vi "GSI-HVSwitch2.initialize interface.vi"(0 "i ref in":refnum<vi>, 3 "ms timeout (10000)":i32=10000, 5 "error in (no error)":errorcluster) -> (14 "i ref out":refnum<vi>, 17 "timed out":bool, 19 "error out":errorcluster)   [LabVIEW 2014, in "GSI-HVSwitch2.lvlib"]
doc: "Initializes the interface to the instrument. This method must be called prior to communicating with the instrument.\n\nLicense Agreement for this software:\n\nCopyright (C)\nGesellschaft für Schwerionenforschung, GSI\nPlanckstr. 1\n64291 Darmstadt\nGermany\n\nContact: D.Beck@gsi.de \n\nThis program is free software; you can redistribute it and/or modify it under the terms of the GNU General Public License as published by the Free Software Foundation; either version 2 of the license, or (at your option) any later version.\n\nThis program is distributed in the hope that it will be useful, but WITHOUT ANY WARRANTY; without even the implied warranty of MERCHANTABILITY or FITNESS FOR A PARTICULAR PURPOSE. See the GNU General License for more details (http://www.gnu.org).\n\nGesellschaft für Schwerionenforschung, GSI\nPlanckstr. 1, 64291 Darmstadt, Germany\nFor all questions and ideas contact: M.Richter@gsi.de, H.Brand@gsi.de or D.Beck@gsi.de.\nLast update: 17-JUN-2004"
uses:
  GSI-HVSwitch2.lvlib
  CSCore/CSApplicationBaseClasses/PSChannelBase/PSChannelBase.myEventNames.ctl
  CSCore/CSApplicationBaseClasses/PSChannelBase/PSChannelBase.directionType.ctl
  CSCore/CSApplicationBaseClasses/PSChannelBase/PSChannelBase.serviceType.ctl
  CSlibraries/UtilityLib/UtilityLib.valueStatus.ctl
  CSCore/CSApplicationBaseClasses/PSChannelBase/PSChannelBase.lvlib
  CSlibraries/UtilityLib/UtilityLib.lvlib
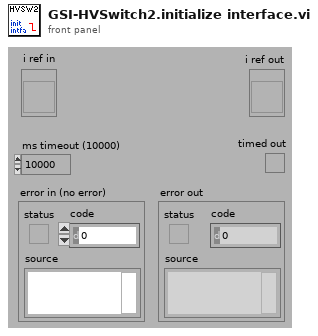
[diagram p1: front panel]
types:
  T1 = typedef "UtilityLib.lvlib/UtilityLib.valueStatus.ctl" = enum16{"no info available", "stand by/off", "on", "warning", "alarm/malfunction", "not implemented", "user action required", "important information", "system default", "control default", "indicator default", "button default"}
  T2 = typedef "PSChannelBase.lvlib/PSChannelBase.serviceType.ctl" = enum16{"onOff", "voltage", "current", "tripCurrent", "rampUpSpeed", "rampDownSpeed", "status"}
  T3 = typedef "PSChannelBase.lvlib/PSChannelBase.directionType.ctl" = enum16{"unknown", "update actual value", "update nominal value", "update both"}
  T4 = typedef "GSI-HVSwitch2.lvlib/GSI-HVSwitch2.i attribute.ctl" = cluster{"SDEX VISA Cluster":T5, "SetVoltage SW0":dbl, "SetVoltage SW1":dbl, "ActTempAmp":dbl, "ActTempPS1":dbl, "ActTempPS2":dbl, "mode":T8, "interfaceInitialized":bool, "serviceIDs":cluster{"nomVoltage0ID":i32, "nomVoltage1ID":i32, "actTempAmpID":i32, "actTempPS1ID":i32, "actTempPS2ID":i32, "modeID":i32}, "usedChannels":i32}
  T5 = typedef "SDEXDriver.lvlib/SDEX.VISA Control.ctl" = cluster{"VISA resource name":refnum<visa-resource-name>, "HEX address":u16, "VISA Timeout Value (1000 ms)":u32, "Lock Timeout (1000 ms)":u32, "semaphore":T6, "Baud rate":u32, "revision":T7, "deviceInfo":string}
  T6 = typedef "Semaphore RefNum" = refnum<k1>
  T7 = typedef "SDEXDriver.lvlib/SDEX.revisionType.ctl" = enum16{"unknown", "hvamp3", "hvswi1", "htrp0", "WDG0"}
  T8 = typedef "GSI-HVSwitch2.lvlib/GSI-HVSwitch2.mode.ctl" = enum16{"unknown", "switch", "stepper"}
  T9 = typedef "PSChannelBase.lvlib/PSChannelBase.myEventNames.ctl" = enum16{"lvmsg://EmergencyOff", "lvmsg://SetOnOff", "lvmsg://GetOnOff", "lvmsg://SetVoltage", "lvmsg://GetVoltage", "lvmsg://SetCurrent", "lvmsg://GetCurrent", "lvmsg://SetTripCurrent", "lvmsg://GetTripCurrent", "lvmsg://SetRampUpSpeed", "lvmsg://GetRampUpSpeed", "lvmsg://SetRampDownSpeed", "lvmsg://GetRampDownSpeed", "lvmsg://SetChannelOnOff", "lvmsg://GetChannelOnOff", "lvmsg://SetChannelVoltage", "lvmsg://GetChannelVoltage", "lvmsg://SetChannelCurrent", "lvmsg://GetChannelCurrent", "lvmsg://SetChannelTripCurrent", "lvmsg://GetChannelTripCurrent", "lvmsg://SetChannelRampUpSpeed", "lvmsg://GetChannelRampUpSpeed", "lvmsg://SetChannelRampDownSpeed", "lvmsg://GetChannelRampDownSpeed"}
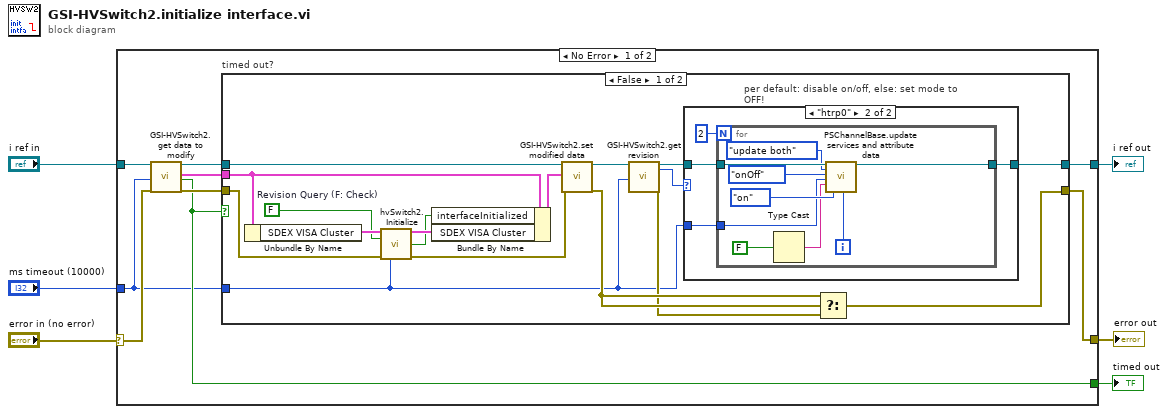
[diagram p0: block diagram]
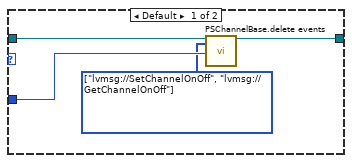
[diagram p2: hidden frame]
diagram:
  n1 = case shown="No Error" "error in (no error)" {
    selector: "error in (no error)" -> [w10 w52]
    tunnel: "i ref in" -> [w15 w53]
    tunnel: [w8 w53] -> w5
    tunnel: [w7 w52] -> w4
    tunnel: [w12 _] -> w3
    tunnel: "ms timeout (10000)" -> [w9 _]
    frame No Error {
      n2 = call "GSI-HVSwitch2.get data to modify.vi"("i ref in"=w15, "ms timeout (10000)"=w9, "error in (no error)"=w10) -> ("i ref out"=w14:refnum<vi>, "i attribute"=w11:T4, "timed out"=w12:bool, "error out"=w13:errorcluster)  [unwired: 13 in]
      n3 = case "timed out?" shown="False" w12 {
        tunnel: [w16 w51] -> w8
        tunnel: w14 -> [w26 w51]
        tunnel: [w20 w50] -> w7
        tunnel: w13 -> [w28 w50]
        tunnel: w11 -> [w31 _]
        tunnel: w9 -> [w17 _]
        frame False {
          w27 = FALSE  # Revision Query (F: Check)
          n4 = Unbundle By Name(w31) -> ("SDEX VISA Cluster"=w32:T5)
          n5 = call "hvSwitch2.Initialize.vi"("SDEX VISA Cluster"=w32, "Revision Query (F: Check)"=w27, "error in (no error)"=w28, "Open timeout (1000ms)"=w17) -> ("dup SDEX VISA Cluster"=w29:T5, "interface initialized"=w25:bool, "error out"=w23:errorcluster)  [unwired: 8 in, 1 out]
          n6 = Bundle By Name(cluster=w31, "interfaceInitialized"=w25, "SDEX VISA Cluster"=w29) -> (w30:T4)
          n7 = call "GSI-HVSwitch2.set modified data.vi"("i ref in"=w26, "i attribute"=w30, "error in (no error)"=w23) -> ("i ref out"=w24:refnum<vi>, "error out"=w22:errorcluster)  [unwired: 15 in]
          n8 = call "GSI-HVSwitch2.get revision.vi"("i ref in"=w24, "ms timeout (10000)"=w17) -> ("i ref out"=w19:refnum<vi>, "revisionType"=w18:T7, "error out"=w21:errorcluster)  [unwired: 13 in, 2 out]
          n9 = case "per default: disable on/off, else: set mode to OFF!" shown="\"htrp0\"" w18 {
            tunnel: w19 -> [w36 w39]
            tunnel: [w35 w40] -> w16
            tunnel: w17 -> [w34 w38]
            frame Default {
              w33 = T9[] [enum."lvmsg://SetChannelOnOff", enum."lvmsg://GetChannelOnOff"] items=["lvmsg://EmergencyOff", "lvmsg://SetOnOff", "lvmsg://GetOnOff", "lvmsg://SetVoltage", "lvmsg://GetVoltage", "lvmsg://SetCurrent", "lvmsg://GetCurrent", "lvmsg://SetTripCurrent", "lvmsg://GetTripCurrent", "lvmsg://SetRampUpSpeed", "lvmsg://GetRampUpSpeed", "lvmsg://SetRampDownSpeed", "lvmsg://GetRampDownSpeed", "lvmsg://SetChannelOnOff", "lvmsg://GetChannelOnOff", "lvmsg://SetChannelVoltage", "lvmsg://GetChannelVoltage", "lvmsg://SetChannelCurrent", "lvmsg://GetChannelCurrent", "lvmsg://SetChannelTripCurrent", "lvmsg://GetChannelTripCurrent", "lvmsg://SetChannelRampUpSpeed", "lvmsg://GetChannelRampUpSpeed", "lvmsg://SetChannelRampDownSpeed", "lvmsg://GetChannelRampDownSpeed"] ("events")
              n10 = call "PSChannelBase.delete events.vi"("i ref in"=w36, "events"=w33, "ms timeout (10000)"=w34) -> ("i ref out"=w35:refnum<vi>)  [unwired: 14 in, 2 out]
            }
            frame "htrp0" {
              n11 = for {
                N: 2 -> [_]
                tunnel: [w41] -> w40
                tunnel: w39 -> [w49]
                tunnel: w38 -> [w44]
                i -> [w42]
                n12 = Type Cast(x=FALSE) -> (*(type *) &x=w45:string)  [unwired: 1 in]
                n13 = call "PSChannelBase.update services and attribute data.vi"("i ref in"=w49, "direction"=PSChannelBase.directionType."update both", "service"=PSChannelBase.serviceType."onOff", "ms timeout (10000)"=w44, "value"=w45, "quality"=UtilityLib.valueStatus."on", "channelNumber"=w42) -> ("i ref out"=w41:refnum<vi>)  [unwired: 10 in, 2 out]
              }
            }
          }
          n14 = Select(t=w22, s=w22, f=w21) -> (s? t:f=w20:errorcluster)
        }
        frame True {
        }
      }
    }
    frame Error {
    }
  }
  "error out" <- w4
  "i ref out" <- w5
  "timed out" <- w3
